vi "DBCreateTableString.vi"() -> (1 "DB Create Table String":string)   [LabVIEW 2015]
uses:
  MainController.lvlib
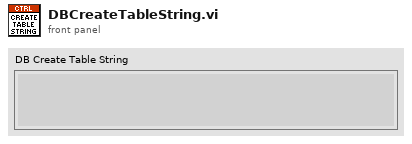
[diagram p1: front panel]
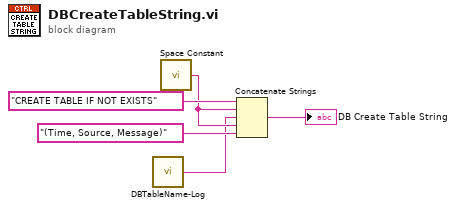
[diagram p0: block diagram]
diagram:
  n1 = call "DBTableName-Log.vi"() -> ("DB Table Name"=w1:string)  [unwired: 5 in]
  n2 = call <vilib>:"Space Constant.vi"() -> ("String"=w3:string)
  n3 = Concatenate Strings("CREATE TABLE IF NOT EXISTS" ("string"), w3, w1, w3, "(Time, Source, Message)" ("string")) -> (→"DB Create Table String":string)
